vi "DISP_WIND_TABL.vi"(0 "VISA IN":refnum<visa-resource-name>, 1 "Tables":string(combo)="SEGMent", 5 "error in":errorcluster, 7 "Window":i32=1) -> (14 "VISA Out":refnum<visa-resource-name>, 19 "error out":errorcluster)   [LabVIEW 2018, in "PNA-X.lvlib"]
doc: "DISPlay:WINDow<wnum>:TABLe <char> \n1593\n\n(Read-Write) Write to show the specified table at the bottom of the analyzer screen or Read to \ndetermine what table is visible. \nParameters \n<wnum> Any existing window number. If unspecified, value is set to 1 \n<char> Table to show. Choose from: \nOFF | MARKer | LIMit | SEGMent \nExamples DISP:WIND:TABLe SEGM \ndisplay:window:table off \nQuery Syntax DISPlay:WINDow:TABLe? \nDefault OFF"
uses:
  PNA-X.lvlib
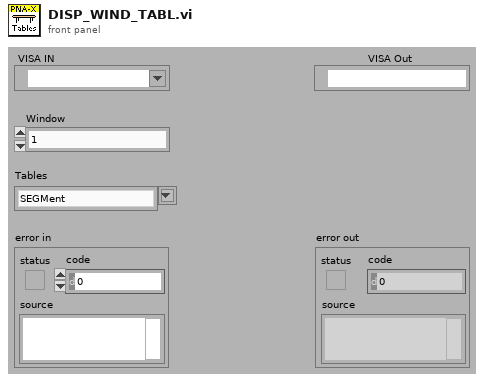
[diagram p1: front panel]
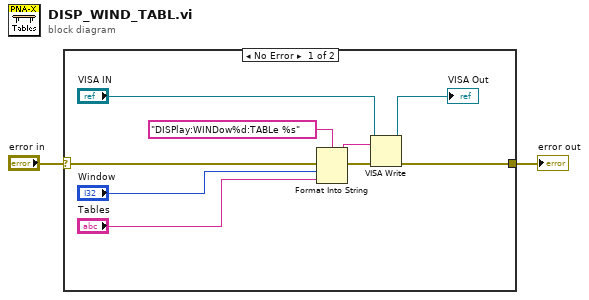
[diagram p0: block diagram]
diagram:
  n1 = case shown="No Error" "error in" {
    selector: "error in" -> [w11 w12]
    tunnel: [w6 w12] -> w1
    frame No Error {
      n2 = Format Into String(format string="DISPlay:WINDow%d:TABLe %s" ("Cmdline"), error in=w11, "Window", "Tables") -> (resulting string=w9:string, error out=w10:errorcluster)  [unwired: 1 in]
      n3 = VISA Write(VISA resource name="VISA IN", write buffer=w9, error in (no error)=w10) -> (VISA resource name out=→"VISA Out":refnum<visa-resource-name>, error out=w6:errorcluster)  [unwired: 1 out]
    }
    frame Error {
    }
  }
  "error out" <- w1
